vi "Ass-4.vi"() -> ()   [LabVIEW 2024]
panel:
  out "XNOR":bool
  out "XOR":bool
  out "NAND":bool
  out "NOR":bool
  out "NOT":bool
  out "OR":bool
  out "AND":bool
  in  "B":bool
  in  "A":bool
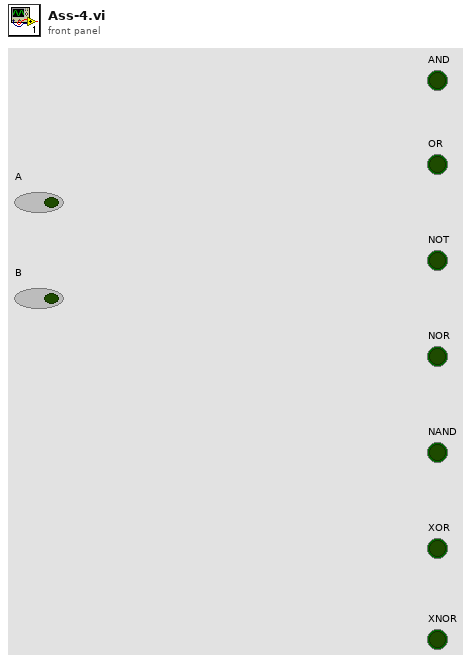
[diagram p1: front panel]
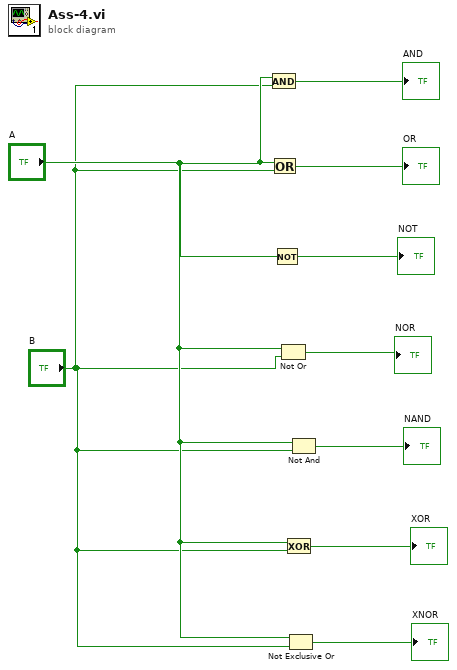
[diagram p0: block diagram]
diagram:
  n1 = And(x="A", y="B") -> (x .and. y?=→"AND":bool)
  n2 = Or(x="A", y="B") -> (x .or. y?=→"OR":bool)
  n3 = Not(x="A") -> (.not. x?=→"NOT":bool)
  n4 = Not Or(1:"B", 2:"A") -> (0:→"NOR":bool)
  n5 = Exclusive Or(1:"B", 2:"A") -> (0:→"XOR":bool)
  n6 = Not Exclusive Or(1:"B", 2:"A") -> (0:→"XNOR":bool)
  n7 = Not And(1:"B", 2:"A") -> (0:→"NAND":bool)
